vi "Array of Variants to Array Variant.vi"(8 "error in (no error)":errorcluster, 11 "[Variant]":variant[](array[variant])) -> (0 "error out":errorcluster, 3 "Array Variant":variant)   [LabVIEW 2018, in "Potentiostat Galvanostat.lvclass"]
uses:
  Potentiostat Galvanostat.lvclass
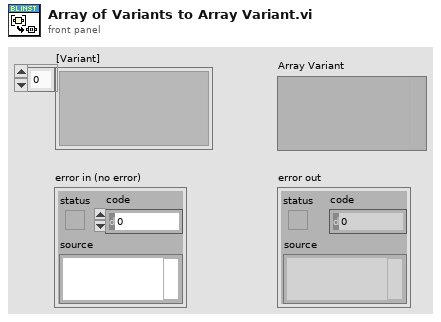
[diagram p1: front panel]
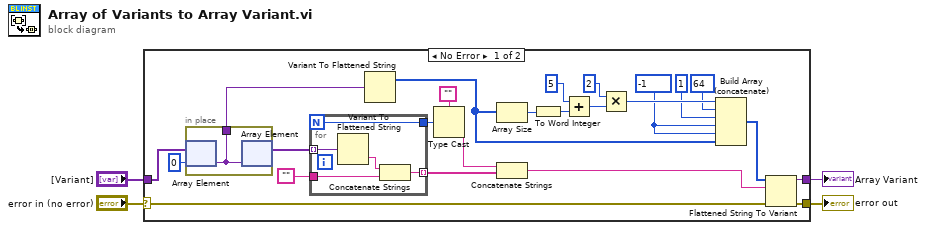
[diagram p0: block diagram]
diagram:
  n1 = case shown="No Error" "error in (no error)" {
    selector: "error in (no error)" -> [w15 w35]
    tunnel: [w14 w35] -> w1
    tunnel: "[Variant]" -> [w8 _]
    tunnel: [w13 _] -> w2
    frame No Error {
      w17 = i16 -1
      n2 = in-place {
        in-place-border: [w29] -> w5
        n3 = in-place-array #1(w8, 0) -> (w29:variant)
        n4 = in-place-array #1(w29) -> (w7:variant[])  [unwired: 1 out]
      }
      n5 = for {
        N -> [w31]
        tunnel: w7 -> [w30] mode=indexing
        tunnel: "" -> [w34]
        tunnel: [w32] -> w27 mode=indexing
        tunnel: [w31] -> w10
        n6 = Variant To Flattened String(Variant=w30) -> (data string=w33:string)  [unwired: 1 out]
        n7 = Concatenate Strings(w33, w34) -> (w32:string)
      }
      n8 = Variant To Flattened String(Variant=w5) -> (1:w11:i16[])  [unwired: 1 out]
      n9 = Type Cast(type="", x=w10) -> (*(type *) &x=w26:string)
      n10 = Array Size(array=w11) -> (size(s)=w25:i32)
      n11 = Concatenate Strings(w26, w27) -> (w12:string)
      n12 = To Word Integer(number=w25) -> (16bit integer=w24:i16)
      n13 = Add(x=i16 5, y=w24) -> (x+y=w22:i16)
      n14 = Multiply(x=i16 2, y=w22) -> (x*y=w20:i16)
      n15 = Build Array (concatenate)(w20, i16 64, i16 1 ("element"), w17, w17, w11) -> (w16:i16[])
      n16 = Flattened String To Variant(4:w15, 6:w12, 7:w16) -> (0:w14:errorcluster, 3:w13:variant)
    }
    frame Error {
    }
  }
  "error out" <- w1
  "Array Variant" <- w2
